vi "runtest format STEPS array string.vi"(6 "sxStationId":string, 7 "POST (empty)":T2, 8 "error in (no error)":errorcluster, 9 "Sequence Steps":T3[](array[typedef]), 10 "Test Step Outputs":T4[](array[typedef]), 11 "Connection Refnum":T1) -> (0 "error out":errorcluster, 2 "STEPS array":string, 3 "Connection Refnum":T1, 5 "POST out":T2)   [LabVIEW 2011]
uses:
  tests/Test Output.ctl
  server/database/Steps/Step Record.ctl
  Addons/internet/utils/keyedarr.llb/Keyed Array.ctl
  SI.LIB/ODBC/SQL Controls/Connection Refnum.ctl
  Addons/internet/utils/strutil.llb/Case Matching.ctl
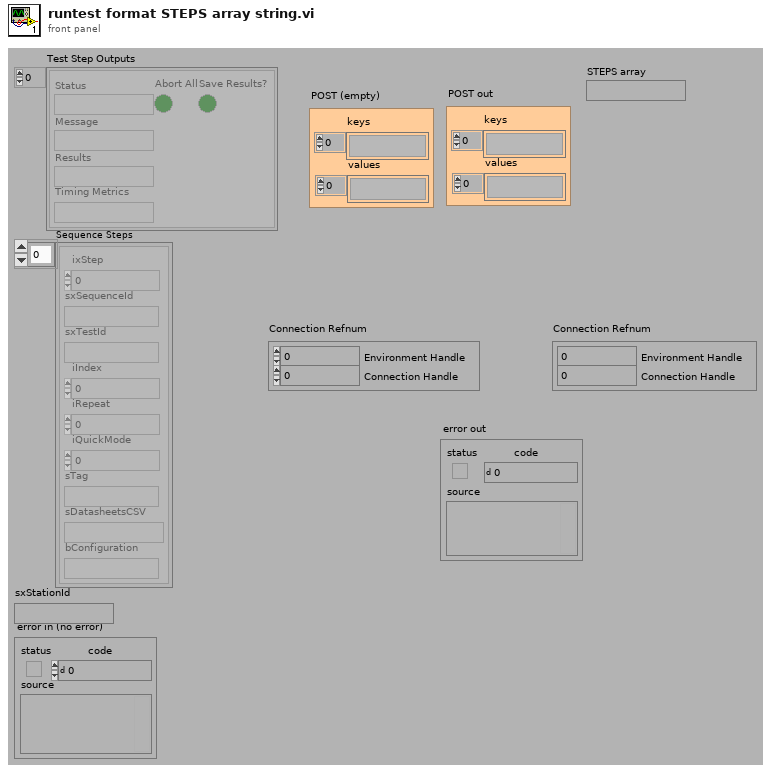
[diagram p1: front panel]
types:
  T1 = typedef "Connection Refnum.ctl" = cluster{"Environment Handle":i32, "Connection Handle":i32}
  T2 = typedef "Keyed Array.ctl" = cluster{"keys":string[], "values":string[]}
  T3 = typedef "Step Record.ctl" = cluster{"ixStep":i32, "sxSequenceId":string, "sxTestId":string, "iIndex":i32, "iRepeat":i32, "iQuickMode":i32, "sTag":string, "sDatasheetsCSV":string, "bConfiguration":string}
  T4 = typedef "Test Output.ctl" = cluster{"Status":string, "Message":string, "Results":string, "Abort All":bool, "Save Results?":bool, "Timing Metrics":string}
  T5 = typedef "Case Matching.ctl" = enum16{"a != A", "a == A", "system"}
  T6 = cluster{"Status":string, "Message":string, "Timing":string}
  T7 = cluster{"Status":string, "Message":string, "Timing":string}[]
  T8 = typedef "Station Record.ctl" = cluster{"ixStation":i32, "sxStationId":string, "sIP":string, "fVerified":bool}
  T9 = typedef "Test Record.ctl" = cluster{"ixTest":i32, "sxTestId":string, "sVersion":string, "sDriverTypes":string[], "sDescription":string, "iQuickMode":i32}
  T10 = typedef "Step Association Record.ctl" = cluster{"ixStepAssociation":i32, "iStep":i32, "iStation":i32, "iInstrument":i32}
  T11 = typedef "Instrument Record.ctl" = cluster{"ixInstrument":i32, "sxInstrumentId":string, "sDriverId":string, "sDriverType":string, "sSerialNumber":string, "tLastCalibration":timestamp, "tCalibrationDue":timestamp, "sConfiguration":string}
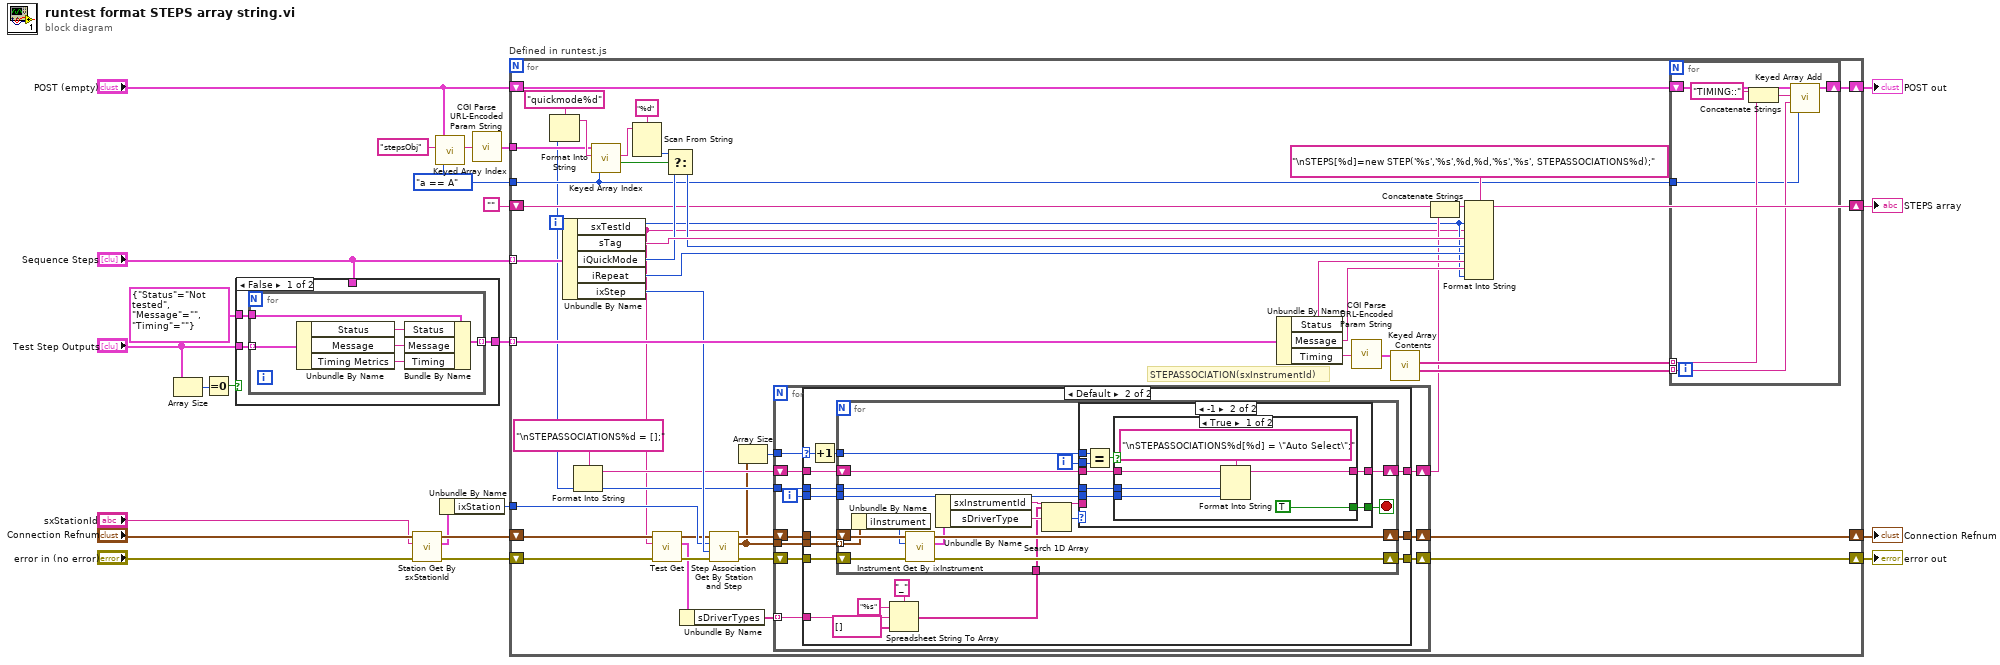
[diagram p0: block diagram]
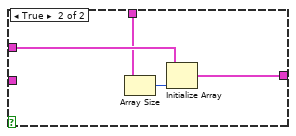
[diagram p2: hidden frame]
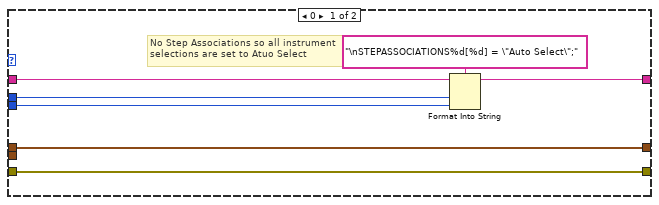
[diagram p3: hidden frame]
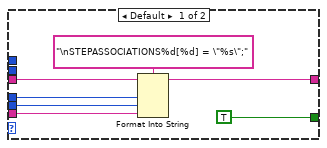
[diagram p4: hidden frame]
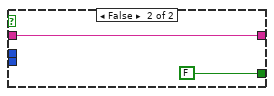
[diagram p5: hidden frame]
diagram:
  w12 = Case_Matching."a == A" ("case matching (sensitive)")
  n1 = Array Size(array="Test Step Outputs") -> (size(s)=w22:i32)
  n2 = Equal To 0?(x=w22) -> (x = 0?=w21:bool)
  n3 = case shown="False" w21 {
    tunnel: T6 {"Status"="Not tested", "Message"="", "Timing"=""} -> [w25 w36]
    tunnel: [w24 w35] -> w19
    tunnel: "Test Step Outputs" -> [w26 _]
    tunnel: "Sequence Steps" -> [_ w33]
    frame False {
      n4 = for {
        tunnel: w26 -> [w32] mode=indexing
        tunnel: w25 -> [w31]
        tunnel: [w30] -> w24 mode=indexing
        n5 = Unbundle By Name(w32) -> ("Status"=w29:string, "Message"=w28:string, "Timing Metrics"=w27:string)
        n6 = Bundle By Name(cluster=w31, "Status"=w29, "Message"=w28, "Timing"=w27) -> (w30:T6)
      }
    }
    frame True {
      n7 = Array Size(array=w33) -> (size(s)=w34:i32)
      n8 = Initialize Array(w36, w34) -> (w35:T7)
    }
  }
  n9 = call "Station Get By sxStationId.vi"("error in (no error)"="error in (no error)", "sxStationId (\"\")"="sxStationId", "Connection Refnum"="Connection Refnum") -> ("error out"=w4:errorcluster, "Station Record"=w2:T8, "Connection Refnum"=w5:T1)  [unwired: 4 in, 2 out]
  n10 = call "Keyed Array Index.vi"("case matching (sensitive)"=w12, "key"="stepsObj", "array in"="POST (empty)") -> ("value"=w14:string)  [unwired: 1 in, 3 out]
  n11 = Unbundle By Name(w2) -> ("ixStation"=w1:i32)
  n12 = call "CGI Parse URL-Encoded Param String.vi"("url-encoded param string"=w14) -> ("params"=w13:T2)
  n13 = for "Defined in runtest.js" {
    tunnel: "Sequence Steps" -> [w81] mode=indexing
    shift-right: [w80] -> w17
    shift-left: "" -> [w48]
    tunnel: w19 -> [w77] mode=indexing
    shift-right: [w70] -> w16
    shift-left: "POST (empty)" -> [w71]
    tunnel: w13 -> [w65]
    tunnel: w12 -> [w58]
    shift-right: [w50] -> w9
    shift-left: w4 -> [w45]
    shift-right: [w51] -> w8
    shift-left: w5 -> [w44]
    tunnel: w1 -> [w56]
    i -> [w46]
    # "STEPASSOCIATION(sxInstrumentId)"
    n14 = Format Into String(format string="quickmode%d" ("key"), w46) -> (resulting string=w67:string)  [unwired: 2 in, 1 out]
    n15 = Unbundle By Name(w81) -> ("sxTestId"=w41:string, "sTag"=w78:string, "iQuickMode"=w60:i32, "iRepeat"=w74:i32, "ixStep"=w57:i32)
    n16 = Format Into String(format string="\nSTEPASSOCIATIONS%d = [];", w46) -> (resulting string=w52:string)  [unwired: 2 in, 1 out]
    n17 = call "Keyed Array Index.vi"("case matching (sensitive)"=w58, "key"=w67, "array in"=w65) -> ("valid key"=w64:bool, "value"=w62:string)  [unwired: 1 in, 2 out]
    n18 = Scan From String(format string="%d", input string=w62) -> (output 1=w61:i32)  [unwired: 2 in, 4 out]
    n19 = call "Test Get.vi"("error in (no error)"=w45, "Test_ID"=w41, "Connection Refnum"=w44) -> ("error out"=w42:errorcluster, "Test Record"=w40:T9, "Connection Refnum"=w43:T1)  [unwired: 5 in, 1 out]
    n20 = Select(t=w61, s=w64, f=w60) -> (s? t:f=w59:i32)
    n21 = Unbundle By Name(w40) -> ("sDriverTypes"=w39:string[])
    n22 = call "Step Association Get By Station and Step.vi"("error in (no error)"=w42, "iStep (0)"=w57, "iStation (0)"=w56, "Connection Refnum"=w43) -> ("error out"=w55:errorcluster, "Step Associations"=w38:T10[], "Connection Refnum"=w54:T1)  [unwired: 4 in, 1 out]
    n23 = Array Size(array=w38) -> (size(s)=w37:i32)
    n24 = for {
      tunnel: w38 -> [w84]
      tunnel: w46 -> [w86]
      shift-right: [w87] -> w49
      shift-left: w52 -> [w90]
      shift-right: [w89] -> w51
      shift-left: w54 -> [w91]
      shift-right: [w88] -> w50
      shift-left: w55 -> [w92]
      tunnel: w39 -> [w85] mode=indexing
      tunnel: w37 -> [w83]
      i -> [w82]
      n25 = case shown="Default" w83 {
        selector: w83 -> [_ w101]
        tunnel: w92 -> [w98 w115]
        tunnel: w91 -> [w99 w114]
        tunnel: w90 -> [w95 w113]
        tunnel: [w99 w112] -> w89
        tunnel: [w98 w111] -> w88
        tunnel: [w96 w110] -> w87
        tunnel: w86 -> [w94 w109]
        tunnel: w85 -> [_ w106]
        tunnel: w84 -> [_ w103]
        tunnel: w82 -> [w93 w100]
        frame 0 {
          # "No Step Associations so all instrument\nselections are set to Atuo Select"
          n26 = Format Into String(format string="\nSTEPASSOCIATIONS%d[%d] = \"Auto Select\";", initial string=w95, w94, w93) -> (resulting string=w96:string)  [unwired: 1 in, 1 out]
        }
        frame Default {
          n27 = Increment(x=w101) -> (x+1=w102:i32)
          n28 = Spreadsheet String To Array(delimiter (Tab)="_", format string="%s" ("delimiter (Tab)"), spreadsheet string=w106, array type (2D Dbl)=string[] []) -> (array=w104:string[])
          n29 = for {
            shift-right: [w132] -> w111
            shift-left: w115 -> [w133]
            shift-right: [w131] -> w112
            shift-left: w114 -> [w130]
            tunnel: w103 -> [w129] mode=indexing
            tunnel: w109 -> [w125]
            shift-right: [w124] -> w110
            shift-left: w113 -> [w123]
            tunnel: w104 -> [w121]
            tunnel: w102 -> [w118]
            tunnel: w100 -> [w117]
            i -> [w116]
            stop <- w119 stop-if-true
            n30 = Unbundle By Name(w129) -> ("iInstrument"=w128:i32)
            n31 = call "Instrument Get By ixInstrument.vi"("error in (no error)"=w133, "ixInstrument"=w128, "Connection Refnum"=w130) -> ("error out"=w132:errorcluster, "Instrument Record"=w127:T11, "Connection Refnum"=w131:T1)  [unwired: 5 in, 1 out]
            n32 = Unbundle By Name(w127) -> ("sxInstrumentId"=w126:string, "sDriverType"=w122:string)
            n33 = Search 1D Array(1D array=w121, element=w122) -> (index of element=w120:i32)  [unwired: 1 in]
            n34 = case shown="-1" w120 {
              tunnel: w126 -> [w139 _]
              tunnel: w117 -> [w138 w144]
              tunnel: w125 -> [w137 w148]
              tunnel: [w136 w147] -> w124
              tunnel: w123 -> [w135 w146]
              tunnel: [TRUE w145] -> w119
              tunnel: w118 -> [_ w142]
              tunnel: w116 -> [_ w141]
              frame Default {
                n35 = Format Into String(format string="\nSTEPASSOCIATIONS%d[%d] = \"%s\";", initial string=w135, w137, w138, w139) -> (resulting string=w136:string)  [unwired: 1 in, 1 out]
              }
              frame -1 {
                n36 = Equal?(x=w142, y=w141) -> (x = y?=w143:bool)
                n37 = case shown="True" w143 {
                  tunnel: w144 -> [w153 _]
                  tunnel: w148 -> [w152 _]
                  tunnel: [w151 w155] -> w147
                  tunnel: w146 -> [w150 w155]
                  tunnel: [TRUE FALSE] -> w145
                  frame True {
                    n38 = Format Into String(format string="\nSTEPASSOCIATIONS%d[%d] = \"Auto Select\";", initial string=w150, w152, w153) -> (resulting string=w151:string)  [unwired: 1 in, 1 out]
                  }
                  frame False {
                  }
                }
              }
            }
          }
        }
      }
    }
    n39 = Unbundle By Name(w77) -> ("Status"=w76:string, "Message"=w75:string, "Timing"=w73:string)
    n40 = call "CGI Parse URL-Encoded Param String.vi"("url-encoded param string"=w73) -> ("params"=w72:T2)
    n41 = call "Keyed Array Contents.vi"("array in"=w72) -> ("values"=w68:string[], "keys"=w69:string[])  [unwired: 5 out]
    n42 = Concatenate Strings(w48, w49) -> (w47:string)
    n43 = Format Into String(format string="\nSTEPS[%d]=new STEP('%s','%s',%d,%d,'%s','%s', STEPASSOCIATIONS%d);", initial string=w47, w46, w41, w78, w59, w74, w76, w75, w46) -> (resulting string=w80:string)  [unwired: 1 in, 1 out]
    n44 = for {
      shift-right: [w162] -> w70
      shift-left: w71 -> [w163]
      tunnel: w69 -> [w160] mode=indexing
      tunnel: w68 -> [w158] mode=indexing
      tunnel: w58 -> [w157]
      n45 = Concatenate Strings("TIMING::", w160) -> (w159:string)
      n46 = call "Keyed Array Add.vi"("case matching (sensitive)"=w157, "value"=w158, "key"=w159, "array in"=w163) -> ("array out"=w162:T2)  [unwired: 3 out]
    }
  }
  "STEPS array" <- w17
  "error out" <- w9
  "POST out" <- w16
  "Connection Refnum" <- w8
